vi "robot movel xyz.vi"(0 "robot_id":i32, 7 "参数":T1, 11 "error in (no error)":errorcluster caption="错误输入（无错误）") -> (4 "robot_id out":i32, 8 "function return":i32, 15 "error out":errorcluster caption="错误输出")   [LabVIEW 2018, in "small_scara_interface.lvlib"]
doc: "extern \"C\" __declspec(dllexport) int robot_movel_xyz(int robot_id, float x, float y, float z, float r, float speed);"
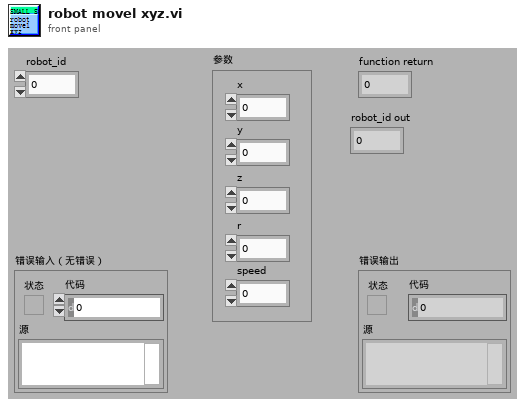
[diagram p1: front panel]
types:
  T1 = cluster{"x":sgl, "y":sgl, "z":sgl, "r":sgl, "speed":sgl}
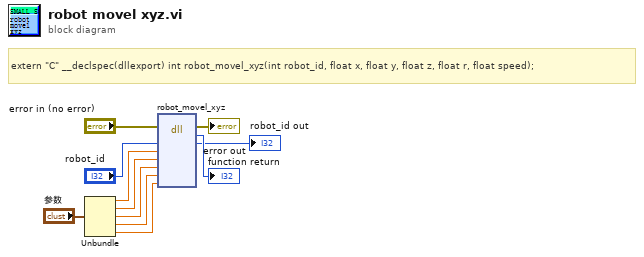
[diagram p0: block diagram]
diagram:
  # "extern \"C\" __declspec(dllexport) int robot_movel_xyz(int robot_id, float x, float y, float z, float r, float speed);"
  n1 = Unbundle("参数") -> ("x"=w6:sgl, "y"=w5:sgl, "z"=w4:sgl, "r"=w3:sgl, "speed"=w2:sgl)
  n2 = dll-call lib="PTH2uabs D测试测试 labview movel_xyzdemo_labview2009Robot-HLsmall_scara_interfacesmall_scara_interface.*" fn="robot_movel_xyz"(error in="error in (no error)", "robot_id"="robot_id", "x"=w6, "y"=w5, "z"=w4, "r"=w3, "speed"=w2) -> (error out=→"error out":errorcluster, "返回类型"=→"function return":i32, "robot_id"=→"robot_id out":i32)  [unwired: 7 in, 1 out]
